vi "StateSpaceUtil_PoseToVector.vi"(11 "Pose":T2={"TRANSLATION"={"X"=0.0, "Y"=0.0}, "ROTATION"={"VALUE"=0.0, "COS"=1.0, "SIN"=0.0}} {"ROTATION"."SIN" format="%13.4f"; "ROTATION"."COS" format="%13.4f"; "ROTATION"."VALUE" format="%13.4f"; "TRANSLATION"."Y" format="%14.3f"; "TRANSLATION"."X" format="%14.3f"}) -> (3 "Pose Vector":T1)   [LabVIEW 2019, in "Trajectory_Library.lvlib"]
doc: "Creates a new LINEAR SYSTEM data cluster with the specified values. \n\n\nInputs: \n - XXX -- XXX.\n\nOutputs:\n - XXX -- XXX."
uses:
  POSE2D.ctl
  TRANSLATION2D.ctl
  ROTATION2D.ctl
  <vilib>/Analysis/Matrix/Datatypes/RealMatrix.ctl
  MatBuilder_Create.vi
  Trajectory_Library.lvlib
  <vilib>/Analysis/Matrix/NI_Matrix.lvlib
panel:
  # "<3,1>"
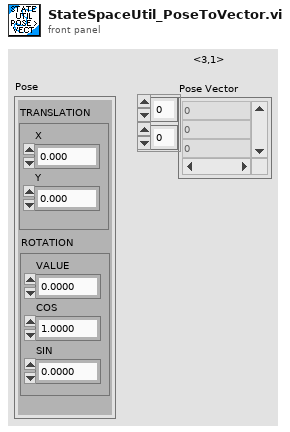
[diagram p1: front panel]
types:
  T1 = typedef "NI_Matrix.lvlib/RealMatrix.ctl" = dbl[][]
  T2 = typedef "Trajectory_Library.lvlib/POSE2D.ctl" = cluster{"TRANSLATION":T3, "ROTATION":T4}
  T3 = typedef "Trajectory_Library.lvlib/TRANSLATION2D.ctl" = cluster{"X":dbl, "Y":dbl}
  T4 = typedef "Trajectory_Library.lvlib/ROTATION2D.ctl" = cluster{"VALUE":dbl, "COS":dbl, "SIN":dbl}
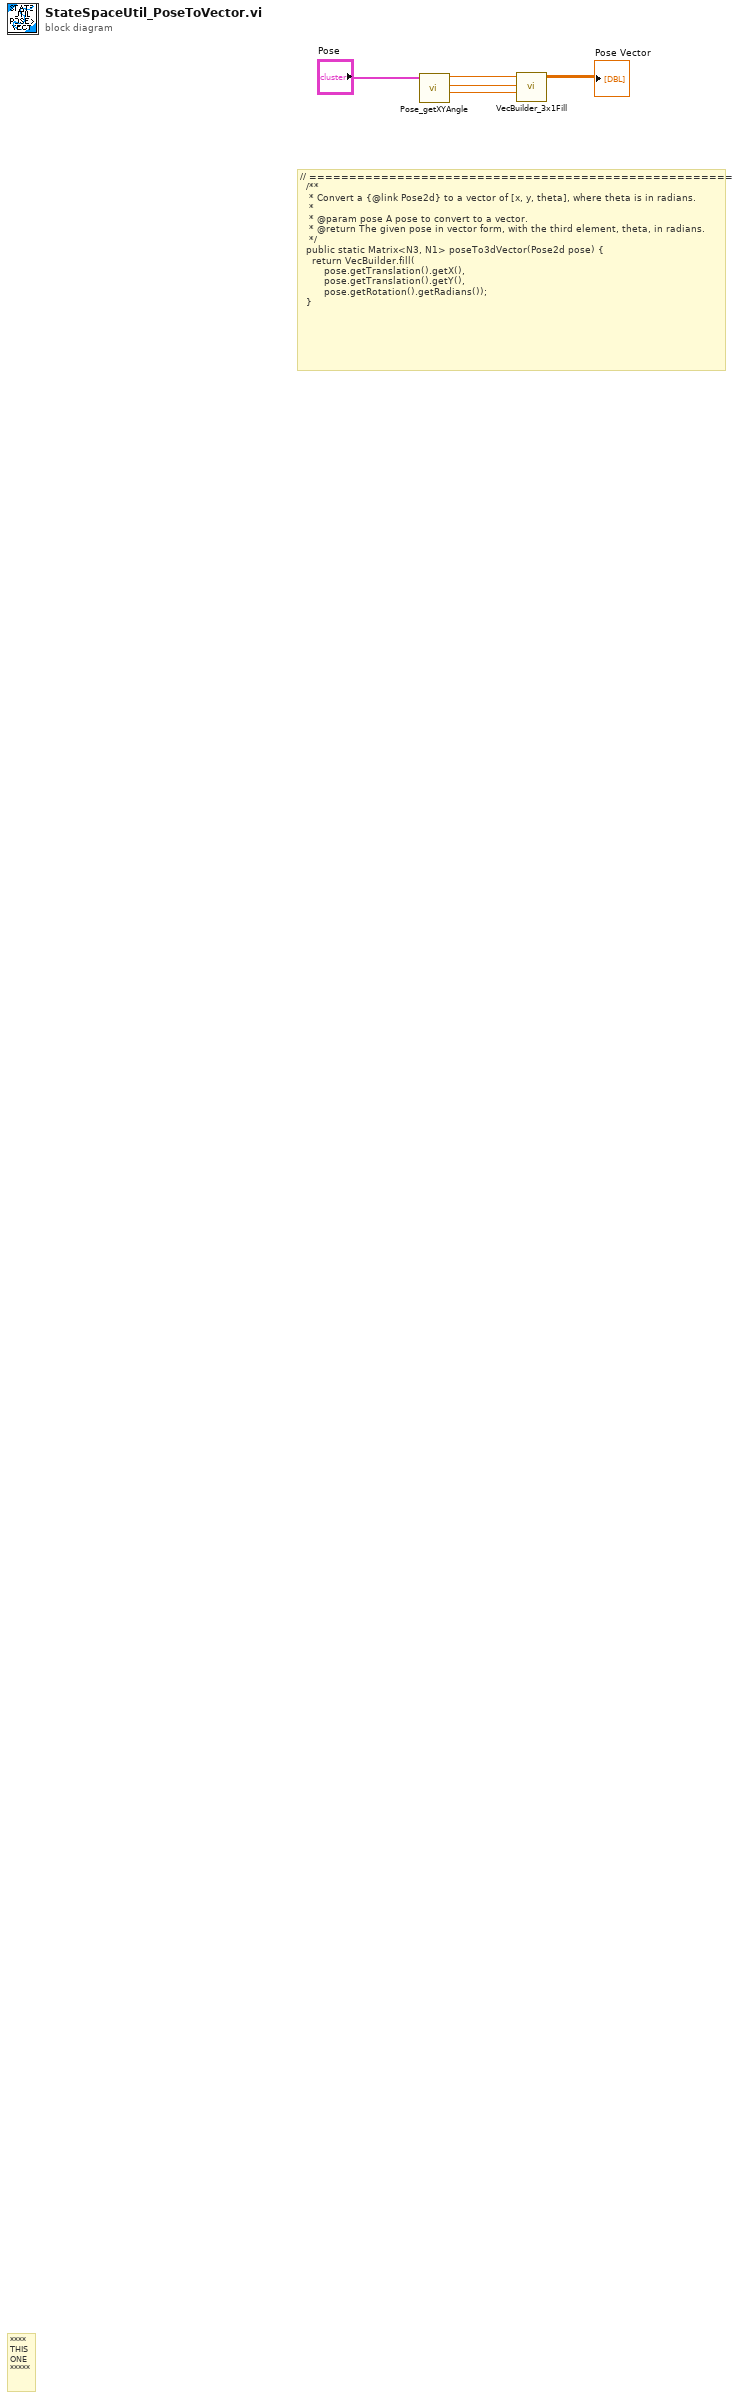
[diagram p0: block diagram]
diagram:
  # "// ======================================================\n  /**\n   * Convert a {@link Pose2d} to a vector of [x, y, theta], where theta is in radians.\n   *\n   * @param pose A pose to convert to a vector.\n   * @return The given pose in vector form, with the third element, theta, in radians.\n   */\n  public static Matrix<N3, N1> poseTo3dVector(Pose2d pose) {\n    return VecBuilder.fill(\n        pose.getTranslation().getX(),\n        pose.getTranslation().getY(),\n        pose.getRotation().getRadians());\n  }"
  # "****\nTHIS\nONE\n*****"
  n1 = call "Pose_getXYAngle.vi"("in POSE"="Pose") -> ("Angle"=w2:dbl, "Y"=w3:dbl, "X"=w4:dbl)  [unwired: 8 in]
  n2 = call "VecBuilder_3x1Fill.vi"("R2"=w2, "R1"=w3, "R0"=w4) -> ("output matrix"=→"Pose Vector":T1)  [unwired: 8 in]
